vi "探头窗口-12-服务器版.vi"() -> ()   [LabVIEW 2013]
panel:
  in  "外部停止命令？":bool=TRUE
  out "引用-探头属性[]":refnum<vi>
  out "引用-监测模式？":refnum<vi>
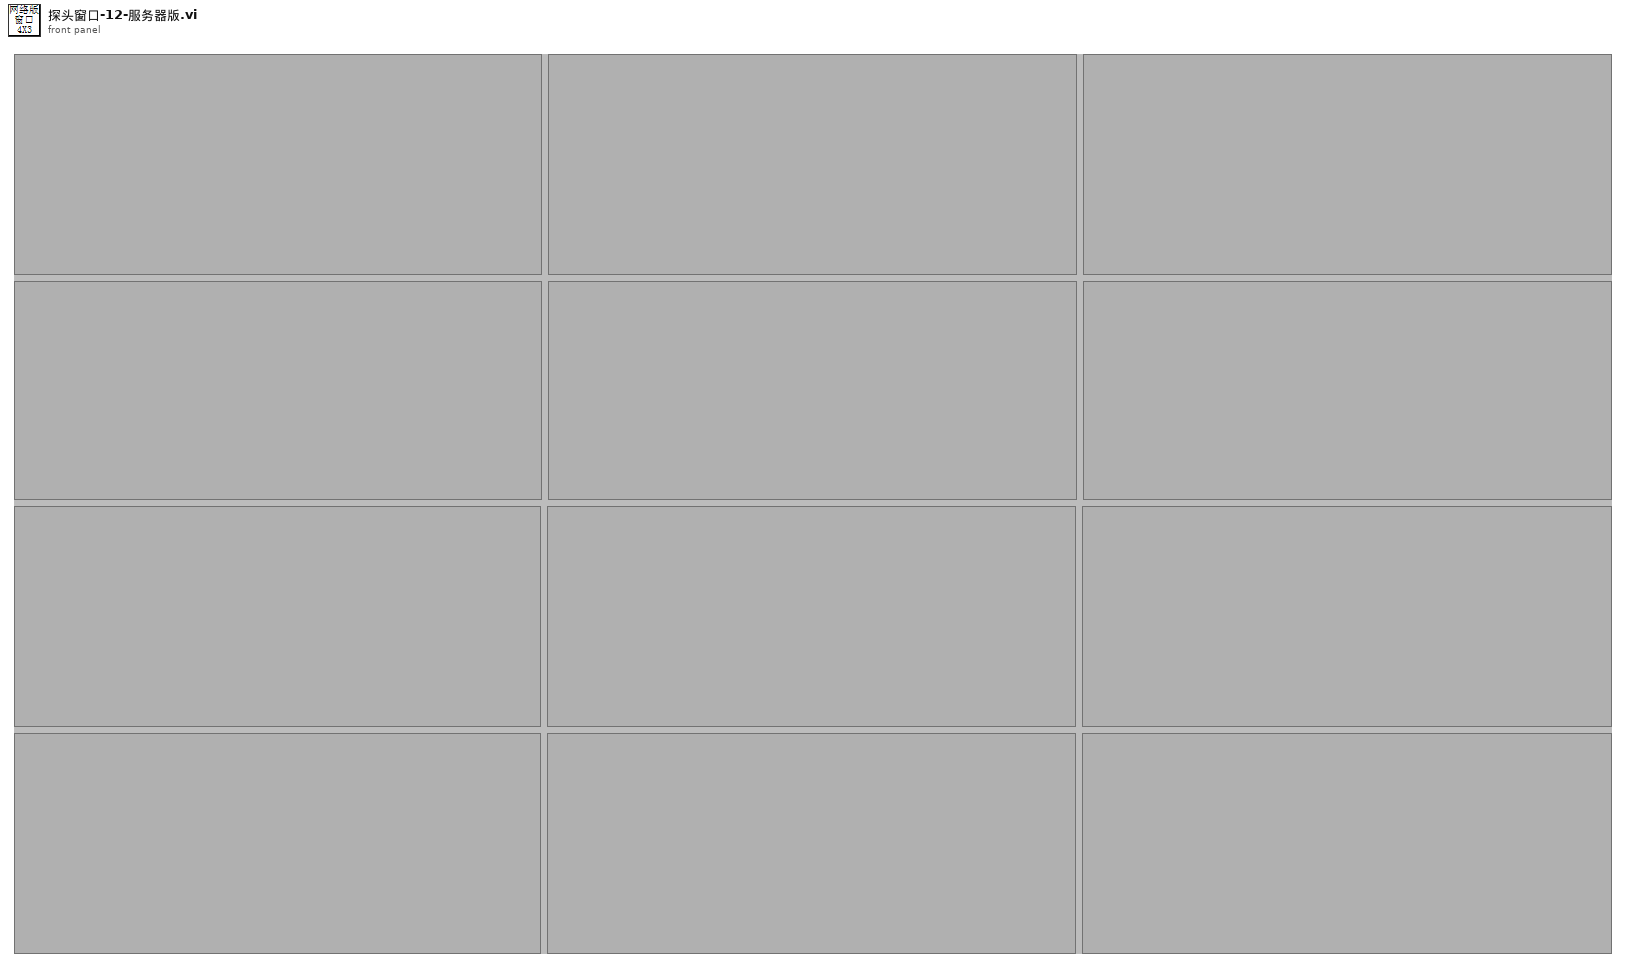
[diagram p1: front panel]
types:
  T1 = typedef "eventvkey.ctl" = enum16{"ASCII", "Enter", "Return", "Shift", "Ctrl", "Alt", "Cmd", "Opt", "Caps", "NumLock", "Clear", "Break", "Up", "Down", "Left", "Right", "Insert", "Delete", "Home", "End", "PageUp", "PageDown", "Escape", "Help", "Pause", "ScrollLock", "F1", "F2", "F3", "F4", "F5", "F6", "F7", "F8", "F9", "F10", "F11", "F12", "F13", "F14", "F15", "F16", "F17", "F18", "F19", "F20", "F21", "F22", "F23", "F24", "Play", "VolumeUp", "VolumeDown", "Mute", "Two Byte Char"}
  T2 = cluster{"探头地址与信息":cluster{"网络地址":cluster{"IP":string, "port":u16}, "探头信息":string}, "测量值":cluster{"时间":timestamp, "数值":dbl}, "限值":cluster{"限值1":dbl, "限值2":dbl}, "探头状态":enum16{"正常", "离线", "禁用", "一级报警", "二级报警"}}[]
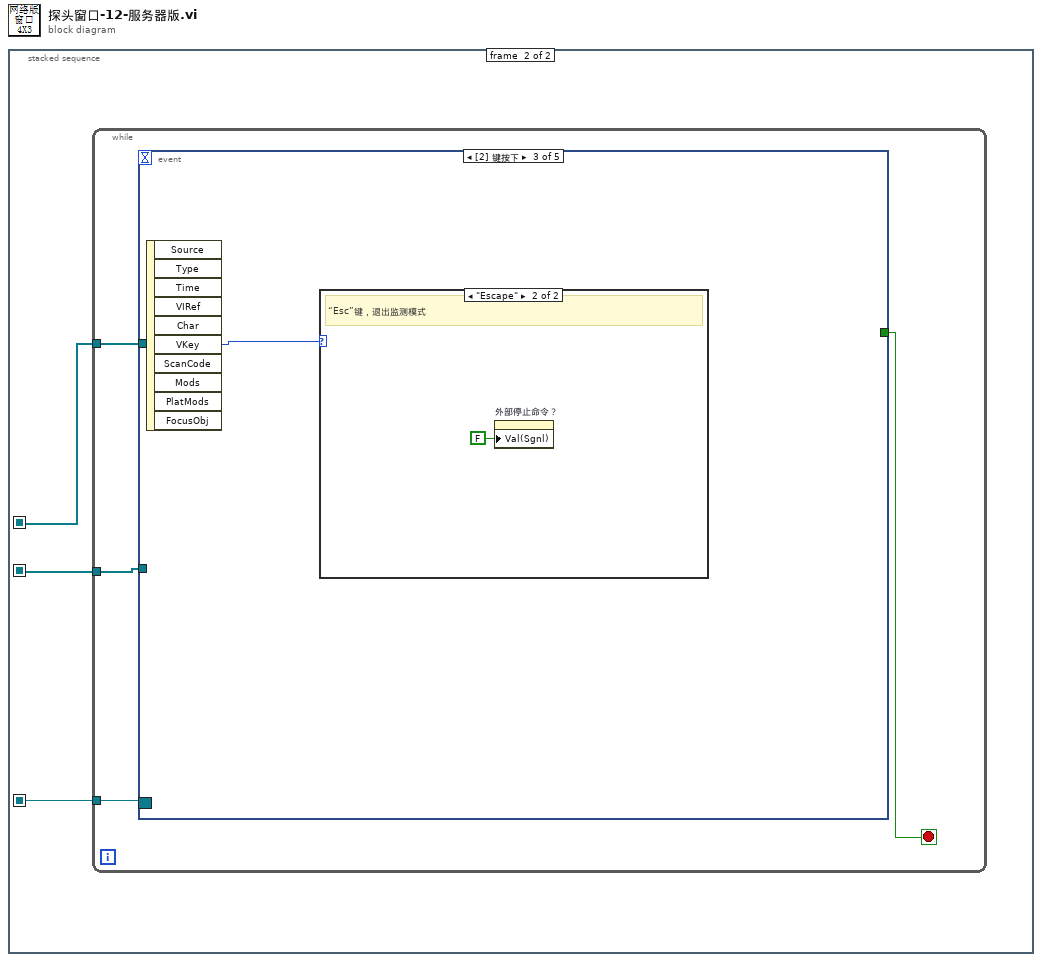
[diagram p0: block diagram]
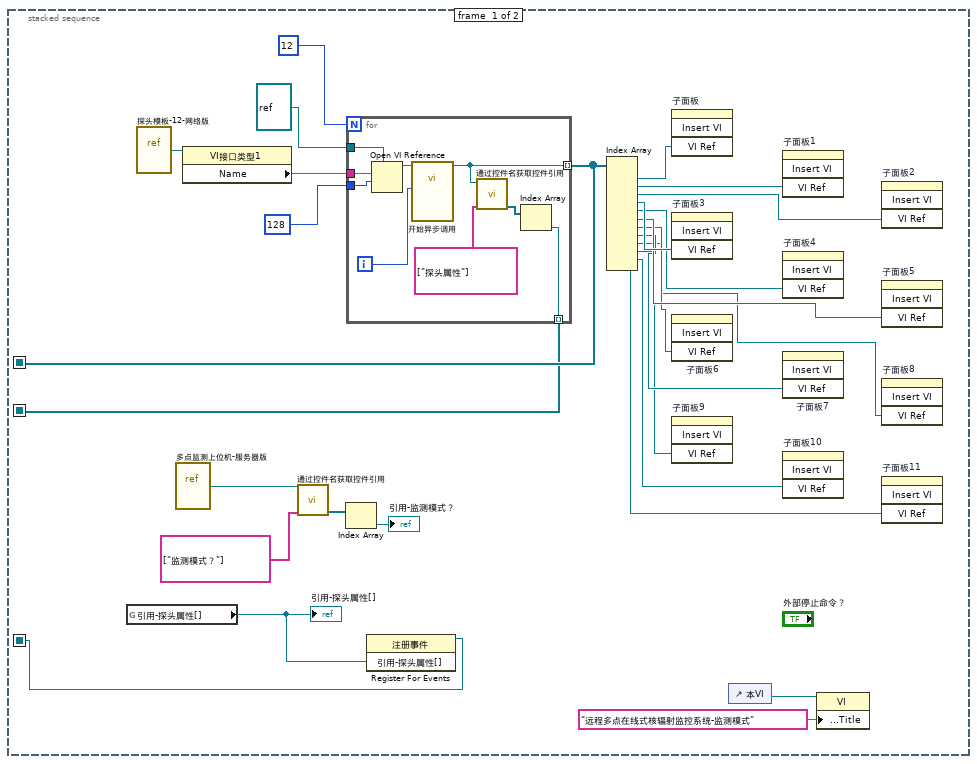
[diagram p2: hidden frame]
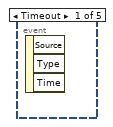
[diagram p3: hidden frame]
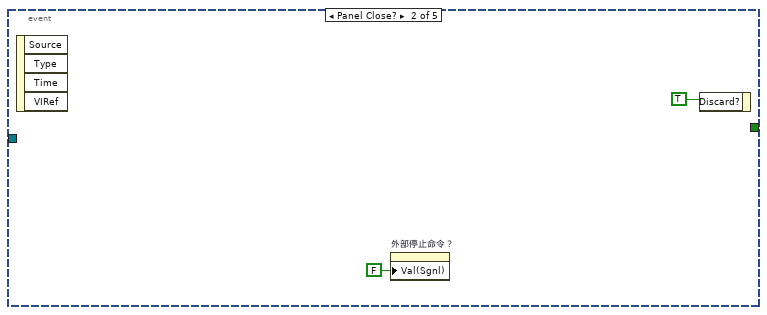
[diagram p4: hidden frame]
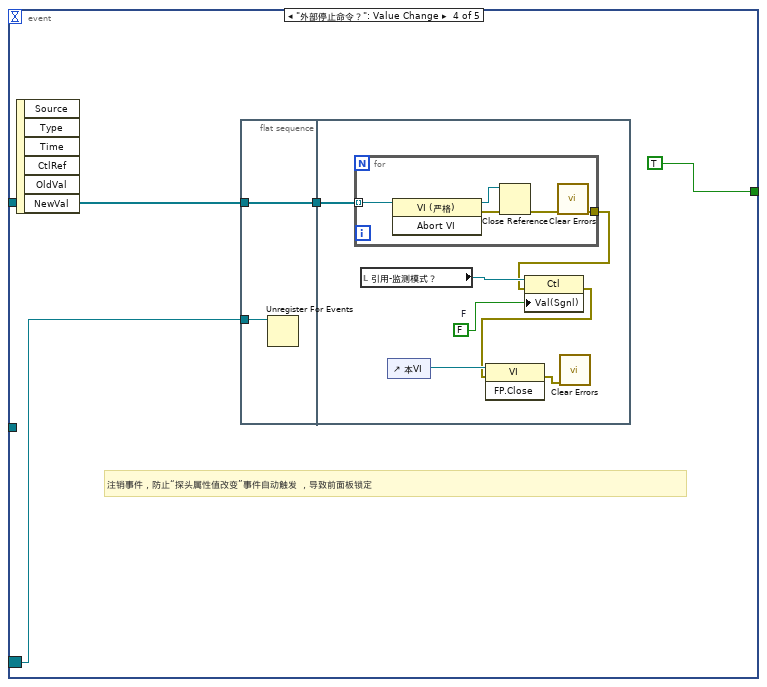
[diagram p6: hidden frame]
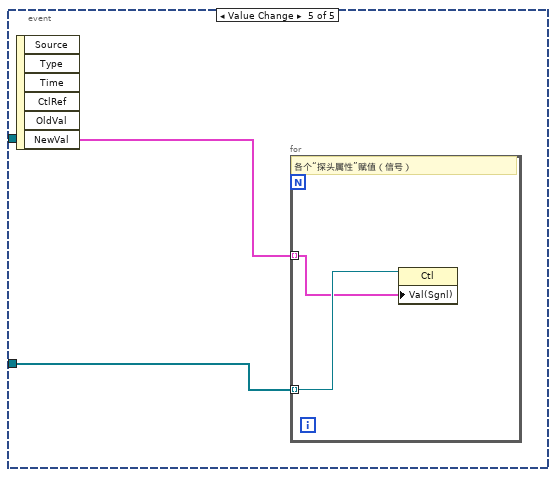
[diagram p7: hidden frame]
diagram:
  n1 = stacked-sequence {
    seq-local: [w23 _] -> [_ w39]
    seq-local: [w21 _] -> [_ w38]
    seq-local: [w3 _] -> [_ w37]
    frame #0 {
      n2 = global read "全局变量-35点监测.vi" "引用-探头属性[]"() -> (w4:refnum<vi>)
      "引用-探头属性[]" <- w4
      n3 = vi-ref "探头模板-12-网络版.vi"() -> (w27:refnum<vi>)
      n4 = vi-ref "多点监测上位机-服务器版.vi"() -> (w5:refnum<vi>)
      n5 = property class="VI接口类型1"(reference=w27) -> ("Name"=w26:string)  [unwired: 1 in, 2 out]
      n6 = call "通过控件名获取控件引用.vi"("控件名数组"=string[] ["监测模式？"], "VI引用"=w5) -> ("控件引用输出"=w7:refnum<vi>[])  [unwired: 7 in, 2 out]
      n7 = Index Array(array=w7) -> (element=→"引用-监测模式？":refnum<vi>)  [unwired: 1 in]
      n8 = for "For循环" {
        N: 12 -> [_]
        tunnel: w26 -> [w36]
        tunnel: 128 ("选项") -> [w35]
        tunnel: refnum<vi> refnum ("类型说明符VI引用句柄（仅用于类型）") -> [w34]
        tunnel: [w29] -> w23 mode=indexing
        tunnel: [w30] -> w21 mode=indexing
        i -> [w28]
        n9 = Open VI Reference(type specifier VI Refnum (for type only)=w34, vi path=w36, options=w35) -> (vi reference=w31:refnum<vi>)  [unwired: 3 in, 1 out]
        n10 = call-by-ref "开始异步调用"(reference=w31, "探头序号"=w28) -> (reference out=w29:refnum<vi>)  [unwired: 12 in, 1 out]
        n11 = call "通过控件名获取控件引用.vi"("控件名数组"=string[] ["探头属性"], "VI引用"=w29) -> ("控件引用输出"=w33:refnum<vi>[])  [unwired: 7 in, 2 out]
        n12 = Index Array(array=w33) -> (element=w30:refnum<vi>)  [unwired: 1 in]
      }
      n13 = register-events(w4) -> (reference out=w3:refnum<event-registration>)  [unwired: 2 in, 1 out]
      n14 = Index Array(array=w23) -> (element #1=w20:refnum<vi>, element #2=w19:refnum<vi>, element #3=w18:refnum<vi>, element #4=w17:refnum<vi>, element #5=w16:refnum<vi>, element #6=w15:refnum<vi>, element #7=w14:refnum<vi>, element #8=w13:refnum<vi>, element #9=w12:refnum<vi>, element #10=w11:refnum<vi>, element #11=w10:refnum<vi>, element #12=w9:refnum<vi>)  [unwired: 12 in]
      n15 = invoke on="子面板" class="子面板" method="Insert VI"("VI Ref"=w20) -> ()  [unwired: 3 in, 4 out]
      n16 = invoke on="子面板3" class="SubPnl" method="Insert VI"("VI Ref"=w17) -> ()  [unwired: 3 in, 4 out]
      n17 = invoke on="子面板6" class="SubPnl" method="Insert VI"("VI Ref"=w14) -> ()  [unwired: 3 in, 4 out]
      n18 = invoke on="子面板9" class="SubPnl" method="Insert VI"("VI Ref"=w11) -> ()  [unwired: 3 in, 4 out]
      n19 = control-ref of="本VI"() -> (w2:refnum<vi>)
      n20 = invoke on="子面板1" class="SubPnl" method="Insert VI"("VI Ref"=w19) -> ()  [unwired: 3 in, 4 out]
      n21 = invoke on="子面板4" class="SubPnl" method="Insert VI"("VI Ref"=w16) -> ()  [unwired: 3 in, 4 out]
      n22 = invoke on="子面板7" class="SubPnl" method="Insert VI"("VI Ref"=w13) -> ()  [unwired: 3 in, 4 out]
      n23 = invoke on="子面板10" class="SubPnl" method="Insert VI"("VI Ref"=w10) -> ()  [unwired: 3 in, 4 out]
      n24 = property class="VI"(reference=w2, "Front Panel.Title"="远程多点在线式核辐射监控系统-监测模式" ("前面板窗口:标题")) -> ()  [unwired: 1 in, 2 out]
      n25 = invoke on="子面板2" class="SubPnl" method="Insert VI"("VI Ref"=w18) -> ()  [unwired: 3 in, 4 out]
      n26 = invoke on="子面板5" class="SubPnl" method="Insert VI"("VI Ref"=w15) -> ()  [unwired: 3 in, 4 out]
      n27 = invoke on="子面板8" class="SubPnl" method="Insert VI"("VI Ref"=w12) -> ()  [unwired: 3 in, 4 out]
      n28 = invoke on="子面板11" class="SubPnl" method="Insert VI"("VI Ref"=w9) -> ()  [unwired: 3 in, 4 out]
    }
    frame #1 {
      n29 = while {
        tunnel: w39 -> [w42]
        tunnel: w38 -> [w41]
        tunnel: w37 -> [w40]
        stop <- w43 stop-if-true
        n30 = event shown="[2] 键按下" {
          selector: w40 -> [_ _ _ w48 _]
          dyn-events: _ -> [_ _ _ _ _]
          timeout: _ -> [_ _ _ _ _]
          tunnel: [_ _ _ TRUE ("放弃？") _] -> w43
          tunnel: w42 -> [_ _ _ w50 _]
          tunnel: w41 -> [_ _ _ _ w66]
          event Timeout {
            n31 = event-data() -> ()  [unwired: 1 in, 3 out]
          }
          event Panel Close? {
            n32 = event-data() -> ()  [unwired: 1 in, 4 out]
            n33 = property on="外部停止命令？" class="Bool (严格)"("Val(Sgnl)"=FALSE ("值(信号)")) -> ()  [unwired: 2 in, 2 out]
            n34 = event-data("Discard?"=TRUE ("放弃？")) -> ()  [unwired: 1 in, 1 out]
          }
          event Key Down {
            n35 = event-data() -> ("VKey"=w46:T1)  [unwired: 1 in, 9 out]
            n36 = case shown="\"Escape\"" w46 {
              frame "ASCII", Default {
              }
              frame "Escape" {
                # "“Esc”键，退出监测模式"
                n37 = property on="外部停止命令？" class="Bool (严格)"("Val(Sgnl)"=FALSE ("值(信号)")) -> ()  [unwired: 2 in, 2 out]
              }
            }
          }
          event "外部停止命令？": Value Change {
            # "注销事件，防止“探头属性值改变”事件自动触发 ，导致前面板锁定"
            n38 = event-data() -> ()  [unwired: 1 in, 6 out]
            n39 = flat-sequence {
              tunnel: w50 -> [w53]
              tunnel: [w53] -> w49
              tunnel: w48 -> [w52]
              tunnel: w49 -> [w60]
              frame #0 {
                n40 = Unregister For Events(event registration refnum=w52) -> ()  [unwired: 1 in, 1 out]
              }
              frame #1 {
                w58 = FALSE  # F
                n41 = for "For循环" {
                  tunnel: w60 -> [w65] mode=indexing
                  tunnel: [w61] -> w56
                  n42 = invoke class="VI (严格)" method="Abort VI"(reference=w65) -> (reference out=w63:refnum<vi>, error out=w64:errorcluster)  [unwired: 2 in, 1 out]
                  n43 = Close Reference(reference=w63, error in (no error)=w64) -> (error out=w62:errorcluster)
                  n44 = call <vilib>:"Clear Errors.vi"("error in (no error)"=w62) -> ("error out"=w61:errorcluster)  [unwired: 6 in]
                }
                n45 = local read "引用-监测模式？"() -> (w59:refnum<vi>)
                n46 = control-ref of="本VI"() -> (w57:refnum<vi>)
                n47 = property class="Ctl"(reference=w59, error in=w56, "Val(Sgnl)"=w58) -> (error out=w55:errorcluster)  [unwired: 1 out]
                n48 = invoke class="VI" method="FP.Close"(reference=w57, error in=w55) -> (error out=w54:errorcluster)  [unwired: 1 in, 2 out]
                n49 = call <vilib>:"Clear Errors.vi"("error in (no error)"=w54) -> ()  [unwired: 6 in, 1 out]
              }
            }
          }
          event Value Change {
            n50 = event-data() -> ("NewVal"=w67:T2)  [unwired: 1 in, 5 out]
            n51 = for "For循环" {
              tunnel: w66 -> [w69] mode=indexing
              tunnel: w67 -> [w68] mode=indexing
              # "各个“探头属性”赋值（信号）"
              n52 = property class="Ctl"(reference=w69, "Val(Sgnl)"=w68) -> ()  [unwired: 1 in, 2 out]
            }
          }
        }
      }
    }
  }
